vi "PWM Set Phase.vi"(9 "pPhase":u16[](array[numeric])=[0, 0, 0, 0, 0, 0, 0, 0], 10 "ChannelMask":u8, 11 "DevHandle":i32) -> (1 "pPhase out":u16[](array[numeric]), 3 "function return":i32)   [LabVIEW 2010, in "usb2pwm.lvlib"]
doc: "int WINAPI PWM_SetPhase(int DevHandle,unsigned char ChannelMask,unsigned short *pPhase);"
uses:
  usb2pwm.lvlib
  USB2XXX/trunk/USB2XXX/USB2XXX/vs2019/Release/USB2XXX.dll
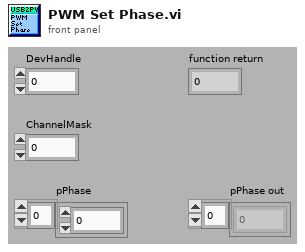
[diagram p1: front panel]
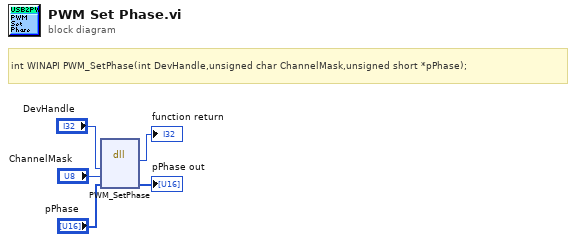
[diagram p0: block diagram]
diagram:
  # "int WINAPI PWM_SetPhase(int DevHandle,unsigned char ChannelMask,unsigned short *pPhase);"
  n1 = dll-call lib="E:/Projects/USB2XXX/trunk/USB2XXX/USB2XXX/vs2019/Release/USB2XXX.*" fn="PWM_SetPhase"("DevHandle"="DevHandle", "ChannelMask"="ChannelMask", "pPhase"="pPhase") -> (→"function return":i32, "pPhase"=→"pPhase out":u16[])  [unwired: 5 in, 2 out]
